vi "Generate_Best_of_Each_DS_Report.vi"(6 "Sort_By":string="Image_AUC", 8 "error in (no error)":errorcluster, 10 "File_Name":string="Best_Of_Each_Dataset.csv", 11 "Destination_Path":path) -> (0 "error out":errorcluster)   [LabVIEW 2020]
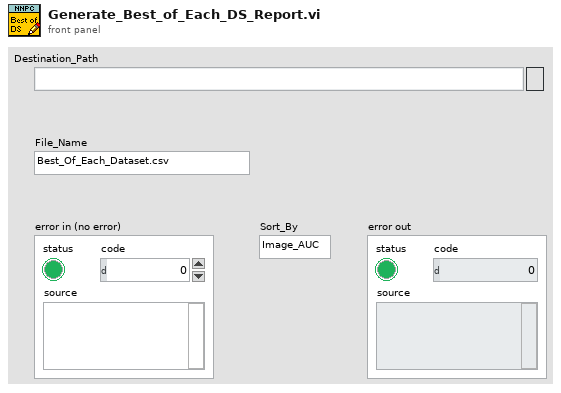
[diagram p1: front panel]
types:
  T1 = enum16{"open", "replace", "create", "open or create", "replace or create", "replace or create with confirmation"}
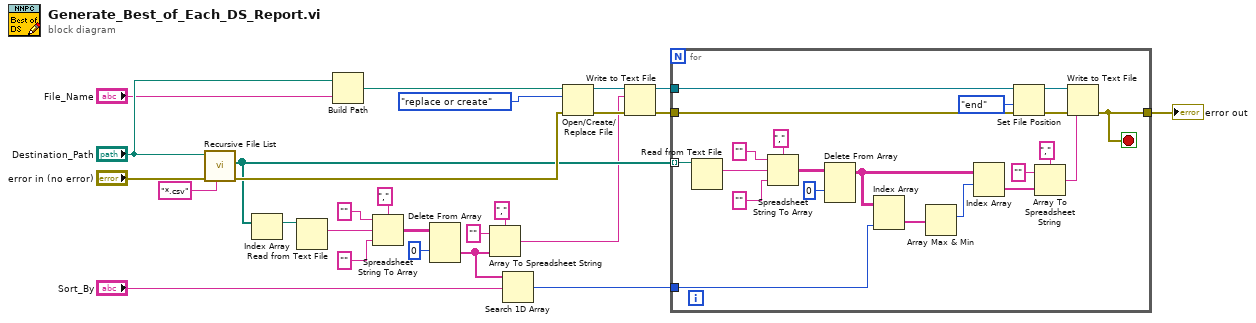
[diagram p0: block diagram]
diagram:
  n1 = call <vilib>:"Recursive File List.vi"("pattern"="*.csv", "error in (no error)"="error in (no error)", "Folder Path"="Destination_Path") -> ("error out"=w18:errorcluster, "All Files in Dir"=w9:path[])  [unwired: 4 in, 3 out]
  n2 = Index Array(array=w9) -> (element=w8:path)  [unwired: 1 in]
  n3 = Read from Text File(file (use dialog)=w8) -> (text=w10:string)  [unwired: 3 in, 3 out]
  n4 = Build Path(base path="Destination_Path", name or relative path="File_Name") -> (appended path=w24:path)
  n5 = Spreadsheet String To Array(delimiter (Tab)=",", format string="", spreadsheet string=w10, array type (2D Dbl)="" ("format string")) -> (array=w14:string[][])
  n6 = Delete From Array(array=w14, index (row)=0) -> (deleted portion=w3:string[])  [unwired: 2 in, 1 out]
  n7 = Array To Spreadsheet String(delimiter (Tab)=",", array=w3, 3:"" ("format string")) -> (spreadsheet string=w5:string)
  n8 = Search 1D Array(1D array=w3, element="Sort_By") -> (index of element=w2:i32)  [unwired: 1 in]
  n9 = Open/Create/Replace File(file path (use dialog)=w24, error in=w18, operation (0:open)=T1."replace or create") -> (refnum out=w23:refnum<file>, error out=w22:errorcluster)  [unwired: 3 in, 1 out]
  n10 = Write to Text File(file (use dialog)=w23, text=w5, error in=w22) -> (refnum out=w16:refnum<file>, error out=w17:errorcluster)  [unwired: 1 in, 1 out]
  n11 = for {
    tunnel: w9 -> [w47] mode=indexing
    tunnel: w17 -> [w34]
    tunnel: w16 -> [w35]
    tunnel: w2 -> [w30]
    tunnel: [w27] -> w1
    stop <- w27 stop-if-true
    n12 = Read from Text File(file (use dialog)=w47) -> (text=w46:string)  [unwired: 3 in, 3 out]
    n13 = Spreadsheet String To Array(delimiter (Tab)=",", format string="", spreadsheet string=w46, array type (2D Dbl)="" ("format string")) -> (array=w42:string[][])
    n14 = Delete From Array(array=w42, index (row)=0) -> (array with subset deleted=w39:string[][])  [unwired: 2 in, 1 out]
    n15 = Index Array(array=w39, index (col)=w30) -> (element=w40:string[])  [unwired: 1 in]
    n16 = Array Max & Min(array=w40) -> (max index (indices)=w38:i32)  [unwired: 3 out]
    n17 = Index Array(array=w39, index (row)=w38) -> (element=w33:string[])  [unwired: 1 in]
    n18 = Set File Position(refnum=w35, from (0:start)=enum16{"start", "end", "current"}."end", error in=w34) -> (refnum out=w37:refnum<file>, error out=w36:errorcluster)  [unwired: 1 in]
    n19 = Array To Spreadsheet String(delimiter (Tab)=",", array=w33, 3:"" ("format string")) -> (spreadsheet string=w28:string)
    n20 = Write to Text File(file (use dialog)=w37, text=w28, error in=w36) -> (error out=w27:errorcluster)  [unwired: 1 in, 2 out]
  }
  "error out" <- w1
